vi "MT_read.vi"(8 "error in (no error)":errorcluster) -> (0 "error out":errorcluster, 3 "Array":dbl[][](array[numeric]))   [LabVIEW 2019]
uses:
  <vilib>/DAQmx/read.llb/DAQmx Read (Analog 2D DBL NChan NSamp).vi
  global_VIs/Global_1.vi
  <vilib>/DAQmx/create/channels.llb/DAQmx Create Channel (AI-Voltage-Basic).vi
  <vilib>/DAQmx/configure/timing.llb/DAQmx Timing (Sample Clock).vi
  <vilib>/DAQmx/miscellaneous.llb/DAQmx Fill In Error Info.vi
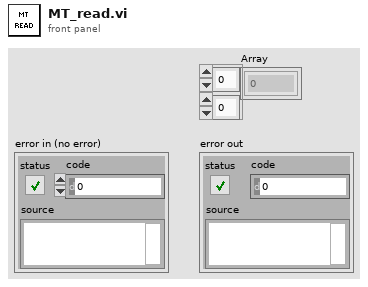
[diagram p1: front panel]
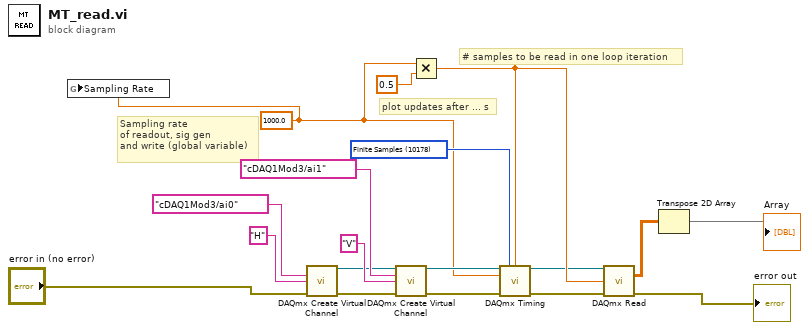
[diagram p0: block diagram]
diagram:
  w11 = 10178 items=["Finite Samples"=10178, "Continuous Samples"=10123, "Hardware Timed Single Point"=12522] ("sample mode")
  w1 = 1000.0 ("rate")
  # "# samples to be read in one loop iteration"
  # "plot updates after ... s"
  # "Sampling rate\nof readout, sig gen\nand write (global variable)"
  n1 = global write "Global_1.vi" "Sampling Rate"(w1) -> ()
  n2 = call-poly <vilib>:"DAQmx Create Virtual Channel.vi"("physical channels"=tag "cDAQ1Mod3/ai0", "name to assign"="H", "error in"="error in (no error)") -> ("task out"=w2:refnum<k21>, "error out"=w3:errorcluster)  [unwired: 11 in]
  n3 = call-poly <vilib>:"DAQmx Create Virtual Channel.vi"("task in"=w2, "physical channels"=tag "cDAQ1Mod3/ai1", "name to assign"="V", "error in"=w3) -> ("task out"=w10:refnum<k21>, "error out"=w9:errorcluster)  [unwired: 10 in]
  n4 = Multiply(x=w1, y=0.5) -> (x*y=w16:dbl)
  n5 = call-poly <vilib>:"DAQmx Timing.vi"("task/channels in"=w10, "sample mode"=w11, "samples per channel"=w16, "rate"=w1, "error in"=w9) -> ("task out"=w12:refnum<k21>, "error out"=w13:errorcluster)  [unwired: 9 in]
  n6 = call-poly <vilib>:"DAQmx Read.vi"("task/channels in"=w12, "number of samples per channel"=w16, "error in"=w13) -> ("data"=w18:dbl[][], "error out"=→"error out":errorcluster)  [unwired: 10 in, 1 out]
  n7 = Transpose 2D Array(2D array=w18) -> (transposed array=→"Array":dbl[][])
